vi "Initialize.vi"(8 "error in (no error)":errorcluster, 11 "GSserver in":refnum<class "GSserver.lvclass">) -> (0 "error out":errorcluster, 3 "GSserver out":refnum<class "GSserver.lvclass">)   [LabVIEW 2018, in "GSserver.lvclass"]
uses:
  GSserver.lvclass
  C:/Users/observer/Desktop/Sparc4GUI/Versao ZeroMQ/SPARC4_GUI - projeto para EXE - 20240702/Server/Server.lvclass
  Server/Server.lvclass/Server.ctl
  Server/Server.lvclass
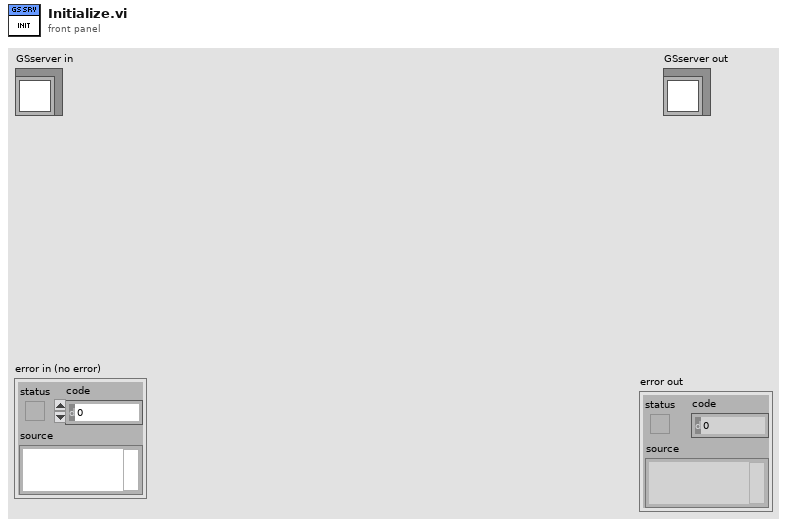
[diagram p1: front panel]
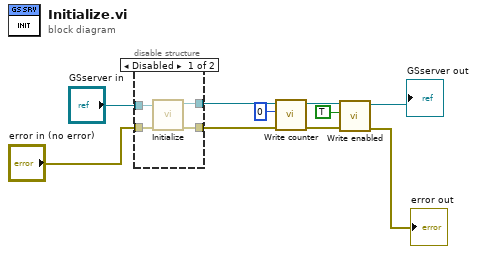
[diagram p0: block diagram]
diagram:
  n1 = disable-structure shown="Disabled" {
    disable-tunnel: [w14 w15] -> w3
    disable-tunnel: [w13 w16] -> w7
    disable-tunnel: "error in (no error)" -> [w12 w15]
    disable-tunnel: "GSserver in" -> [w11 w16]
    frame Disabled {
      n2 = call-parent "Initialize.vi"("error in (no error)"=w12, "Server in"=w11) -> ("error out"=w14:errorcluster, "Server out"=w13:refnum<class "GSserver.lvclass">)  [unwired: 8 in]
    }
    frame Enabled {
    }
  }
  n3 = call "Write counter.vi"("error in (no error)"=w3, "counter"=u32 0, "Server in"=w7) -> ("error out"=w2:errorcluster, "Server out"=w8:refnum<class "GSserver.lvclass">)  [unwired: 7 in]
  n4 = call-dynamic "Write enabled.vi"("error in (no error)"=w2, "enabled"=TRUE, "Server in"=w8) -> ("error out"=→"error out":errorcluster, "Server out"=→"GSserver out":refnum<class "GSserver.lvclass">)  [unwired: 7 in]
